vi "Read Value.vi"(11 "dY_dX_Calculator in":refnum<class "delayValue.lvclass">) -> (1 "oldValue":dbl, 2 "currValue":dbl)   [LabVIEW 2019, in "delayValue.lvclass"]
uses:
  delayValue.lvclass
  delayValue.lvclass/delayValue.ctl
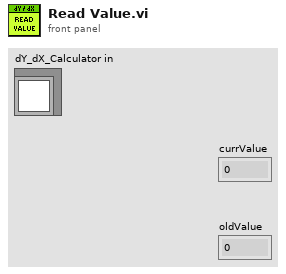
[diagram p1: front panel]
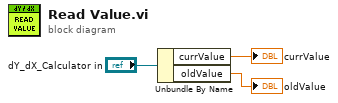
[diagram p0: block diagram]
diagram:
  n1 = Unbundle By Name("dY_dX_Calculator in") -> ("currValue"=→"currValue":dbl, "oldValue"=→"oldValue":dbl)
